vi "check_result_I_calibr.vi"(8 "error_in":errorcluster, 9 "I_control_values":dbl[](array[numeric]), 10 "tolerance_list_I_correction":T1=[{"MIN"="-(0.1+0.01*x*1000)/1000", "MAX"="(0.1+0.01*x*1000)/1000"}, {"MIN"="-(0.1+0.01*x*1000)/1000", "MAX"="(0.1+0.01*x*1000)/1000"}, {"MIN"="-(0.1+0.01*x*1000)/1000", "MAX"="(0.1+0.01*x*1000)/1000"}, {"MIN"="-(0.1+0.01*x*1000)/1000", "MAX"="(0.1+0.01*x*1000)/1000"}, {"MIN"="-(0.1+0.01*x*1000)/1000", "MAX"="(0.1+0.01*x*1000)/1000"}, {"MIN"="-(0.01+0.01*x)", "MAX"="(0.01+0.01*x)"}, {"MIN"="-(0.01+0.01*x)", "MAX"="(0.01+0.01*x)"}, {"MIN"="-(0.01+0.11*x)", "MAX"="(0.01+0.01*x)"}], 11 "result":dbl[][](array[numeric])) -> (0 "error_out":errorcluster, 3 "Array 2":bool[][](array[boolean]))   [LabVIEW 2017]
uses:
  types/tolerance_list.ctl
  types/tolerance.ctl
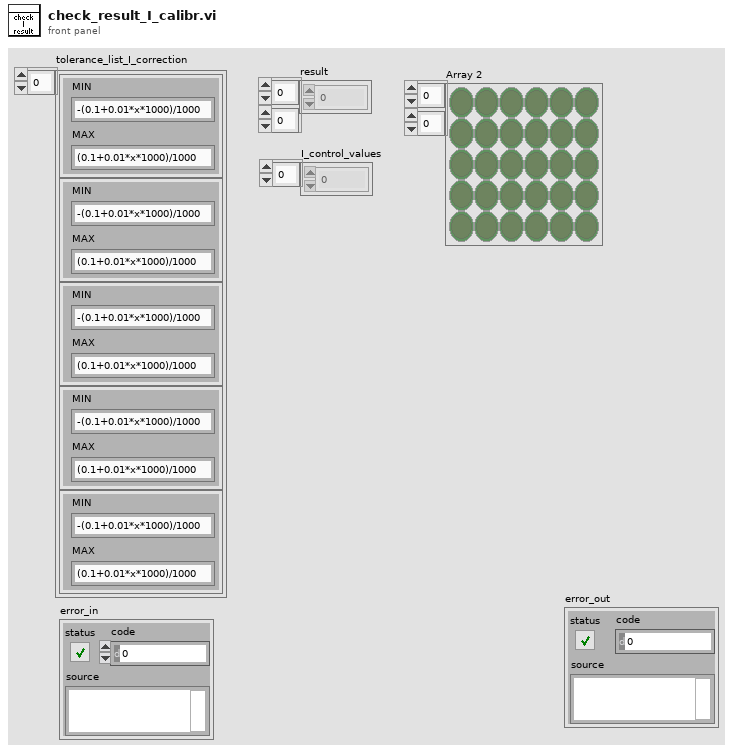
[diagram p1: front panel]
types:
  T1 = typedef "tolerance_list.ctl" = T2[]
  T2 = typedef "tolerance.ctl" = cluster{"MIN":string, "MAX":string}
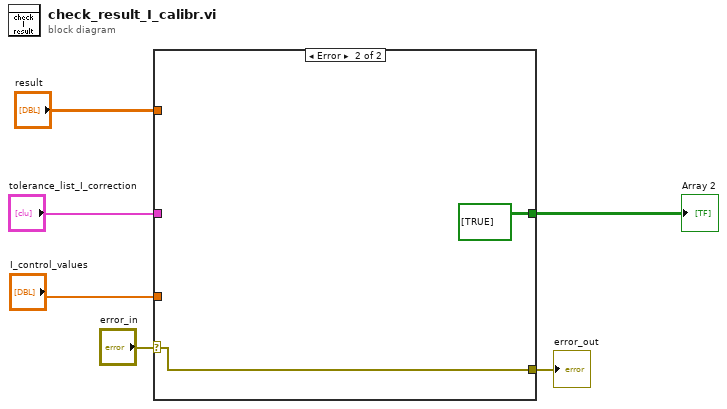
[diagram p0: block diagram]
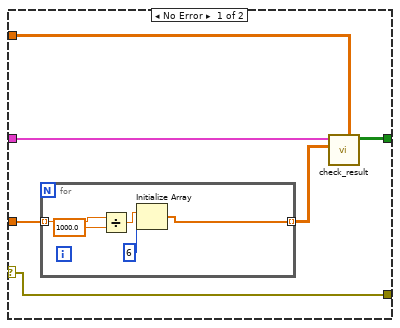
[diagram p2: hidden frame]
diagram:
  n1 = case shown="Error" "error_in" {
    selector: "error_in" -> [w7 w19]
    tunnel: "I_control_values" -> [w12 _]
    tunnel: [w11 bool[][] [[TRUE]] ("Array")] -> w5
    tunnel: "result" -> [w10 _]
    tunnel: "tolerance_list_I_correction" -> [w8 _]
    tunnel: [w7 w19] -> w1
    frame No Error {
      n2 = for {
        tunnel: w12 -> [w15] mode=indexing
        tunnel: [w16] -> w9 mode=indexing
        n3 = Divide(x=w15, y=1000.0) -> (x/y=w13:dbl)
        n4 = Initialize Array(w13, 6 ("dimension size")) -> (w16:dbl[])
      }
      n5 = call "check_result.vi"("RMS"=w10, "measured_value"=w9, "tolerance_list"=w8) -> ("Array"=w11:bool[][])  [unwired: 8 in]
    }
    frame Error {
    }
  }
  "Array 2" <- w5
  "error_out" <- w1
